vi "Adjust the Rock for Chamber.vi"(1 "Chamber Width":i32, 4 "Rock in":u32[][](array[colorbox]), 5 "Rock Distance from Wall":i32, 6 "F: From Left | T: From Right":bool) -> (7 "Rock out":u32[][](array[colorbox]))   [LabVIEW 2020, in "AoC 2022.lvlib"]
uses:
  AoC 2022.lvlib
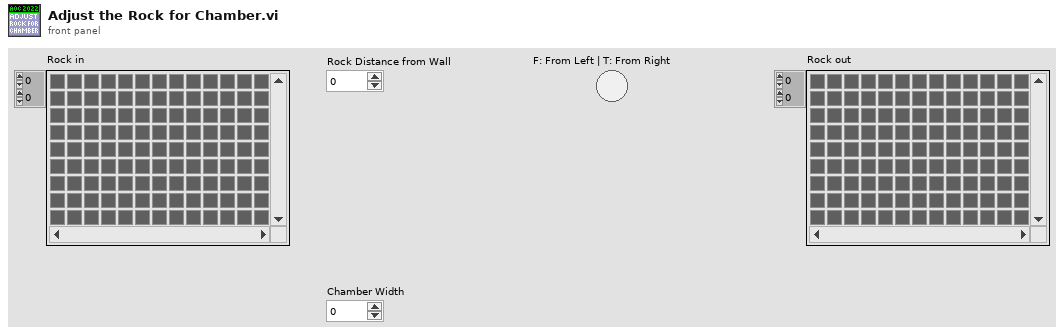
[diagram p1: front panel]
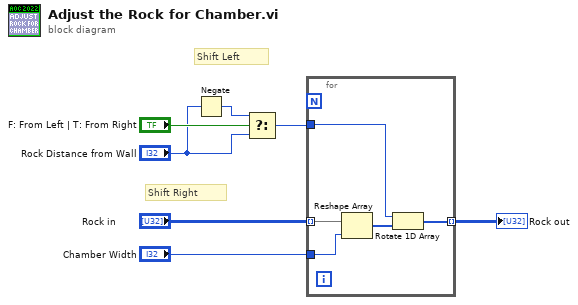
[diagram p0: block diagram]
diagram:
  # "Shift Right"
  # "Shift Left"
  n1 = Negate(x="Rock Distance from Wall") -> (-x=w2:i32)
  n2 = Select(t=w2, s="F: From Left | T: From Right", f="Rock Distance from Wall") -> (s? t:f=w3:i32)
  n3 = for {
    tunnel: [w9] -> w7 mode=indexing
    tunnel: "Rock in" -> [w12] mode=indexing
    tunnel: "Chamber Width" -> [w10]
    tunnel: w3 -> [w8]
    n4 = Reshape Array(w12, w10) -> (w11:u32[])
    n5 = Rotate 1D Array(1:w11, 2:w8) -> (0:w9:u32[])
  }
  "Rock out" <- w7
